vi "Test Camera Module.vi"(8 "error in (no error)":errorcluster) -> (0 "error in (no error) 2":errorcluster)   [LabVIEW 2015]
uses:
  <vilib>/userdefined/High Color/IMAQdx.ctl
  <vilib>/Utility/miscctls.llb/LVPointTypeDef.ctl
  <vilib>/vision/Image Controls.llb/IMAQ Image.ctl
panel:
  out "Status Queue":refnum<queue>
  out "Process Queue":refnum<queue>
  out "Live Queue":refnum<queue>
  in  "Grap image (trigger)":bool
  in  "stop grap":bool
  in  "Grap image":bool
  in  "Camera Connect":bool
  in  "Camera Disconnect":bool
  out "Status log":string
  in  "Camera ID":T1
  in  "Snap Image":bool
  in  "stop":bool
  out "Process Image":T2(plugin-control)
  # "Tests"
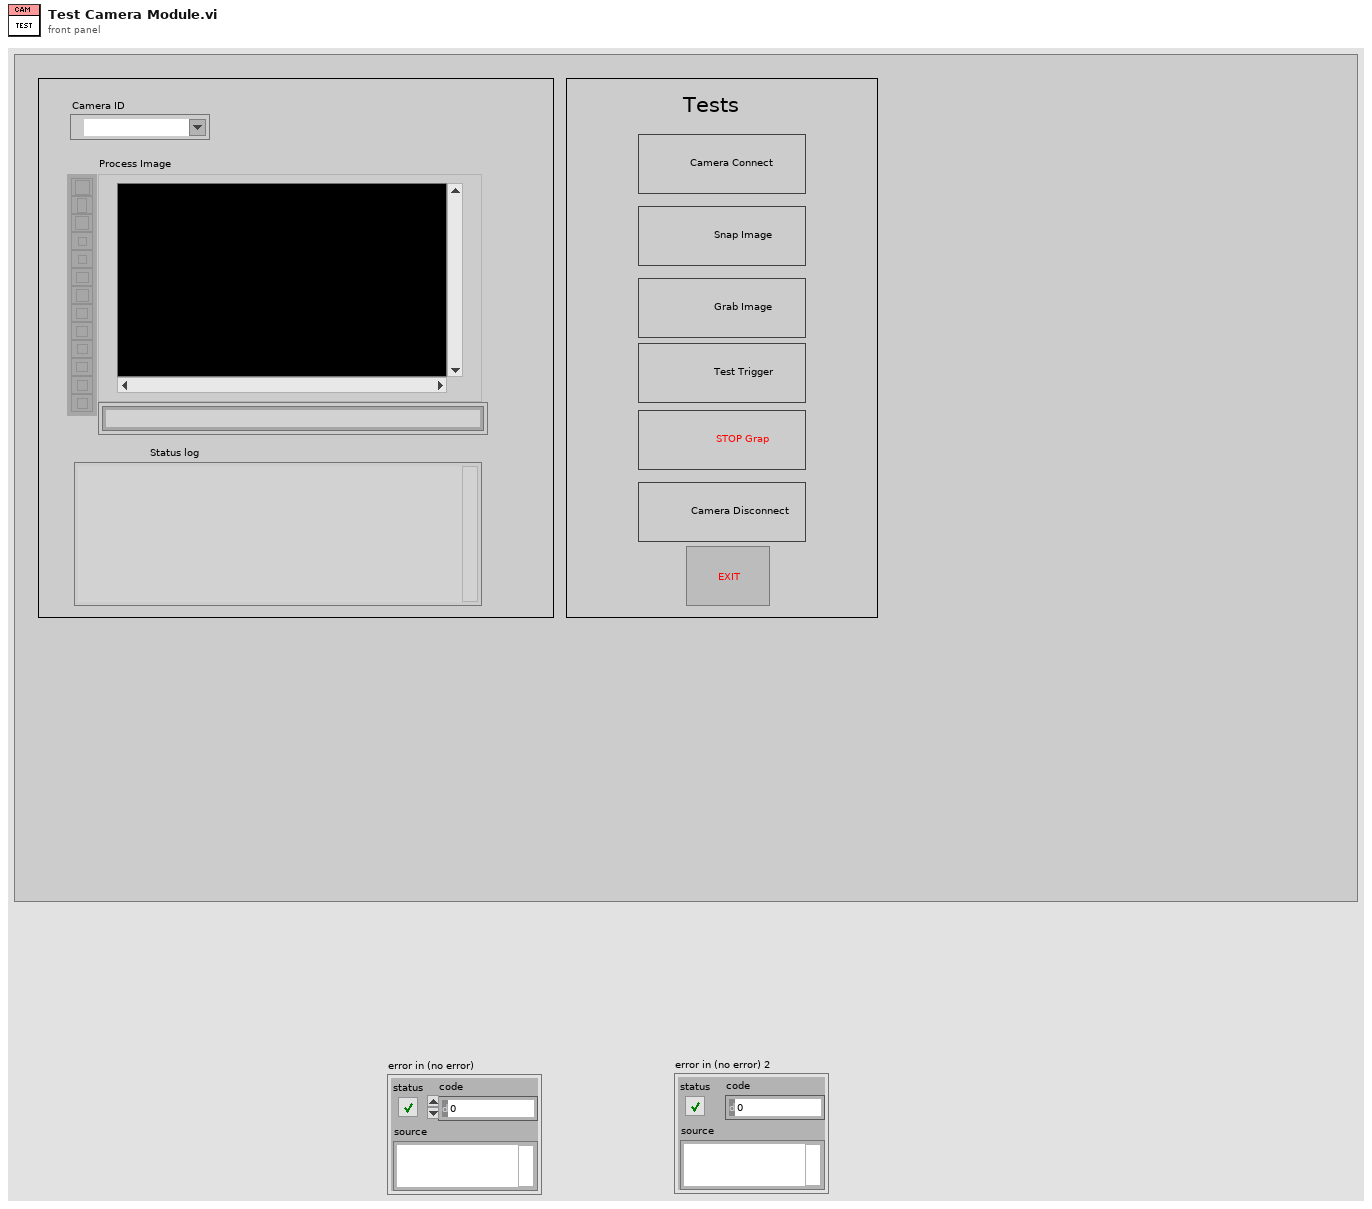
[diagram p1: front panel]
types:
  T1 = typedef "IMAQdx.ctl" = refnum<k21>
  T2 = typedef "IMAQ Image.ctl" = refnum<image>
  T3 = cluster{"Message":string, "Message Data":variant}
  T4 = typedef "LVPointTypeDef.ctl" = cluster{"Horizontal":i16, "Vertical":i16}
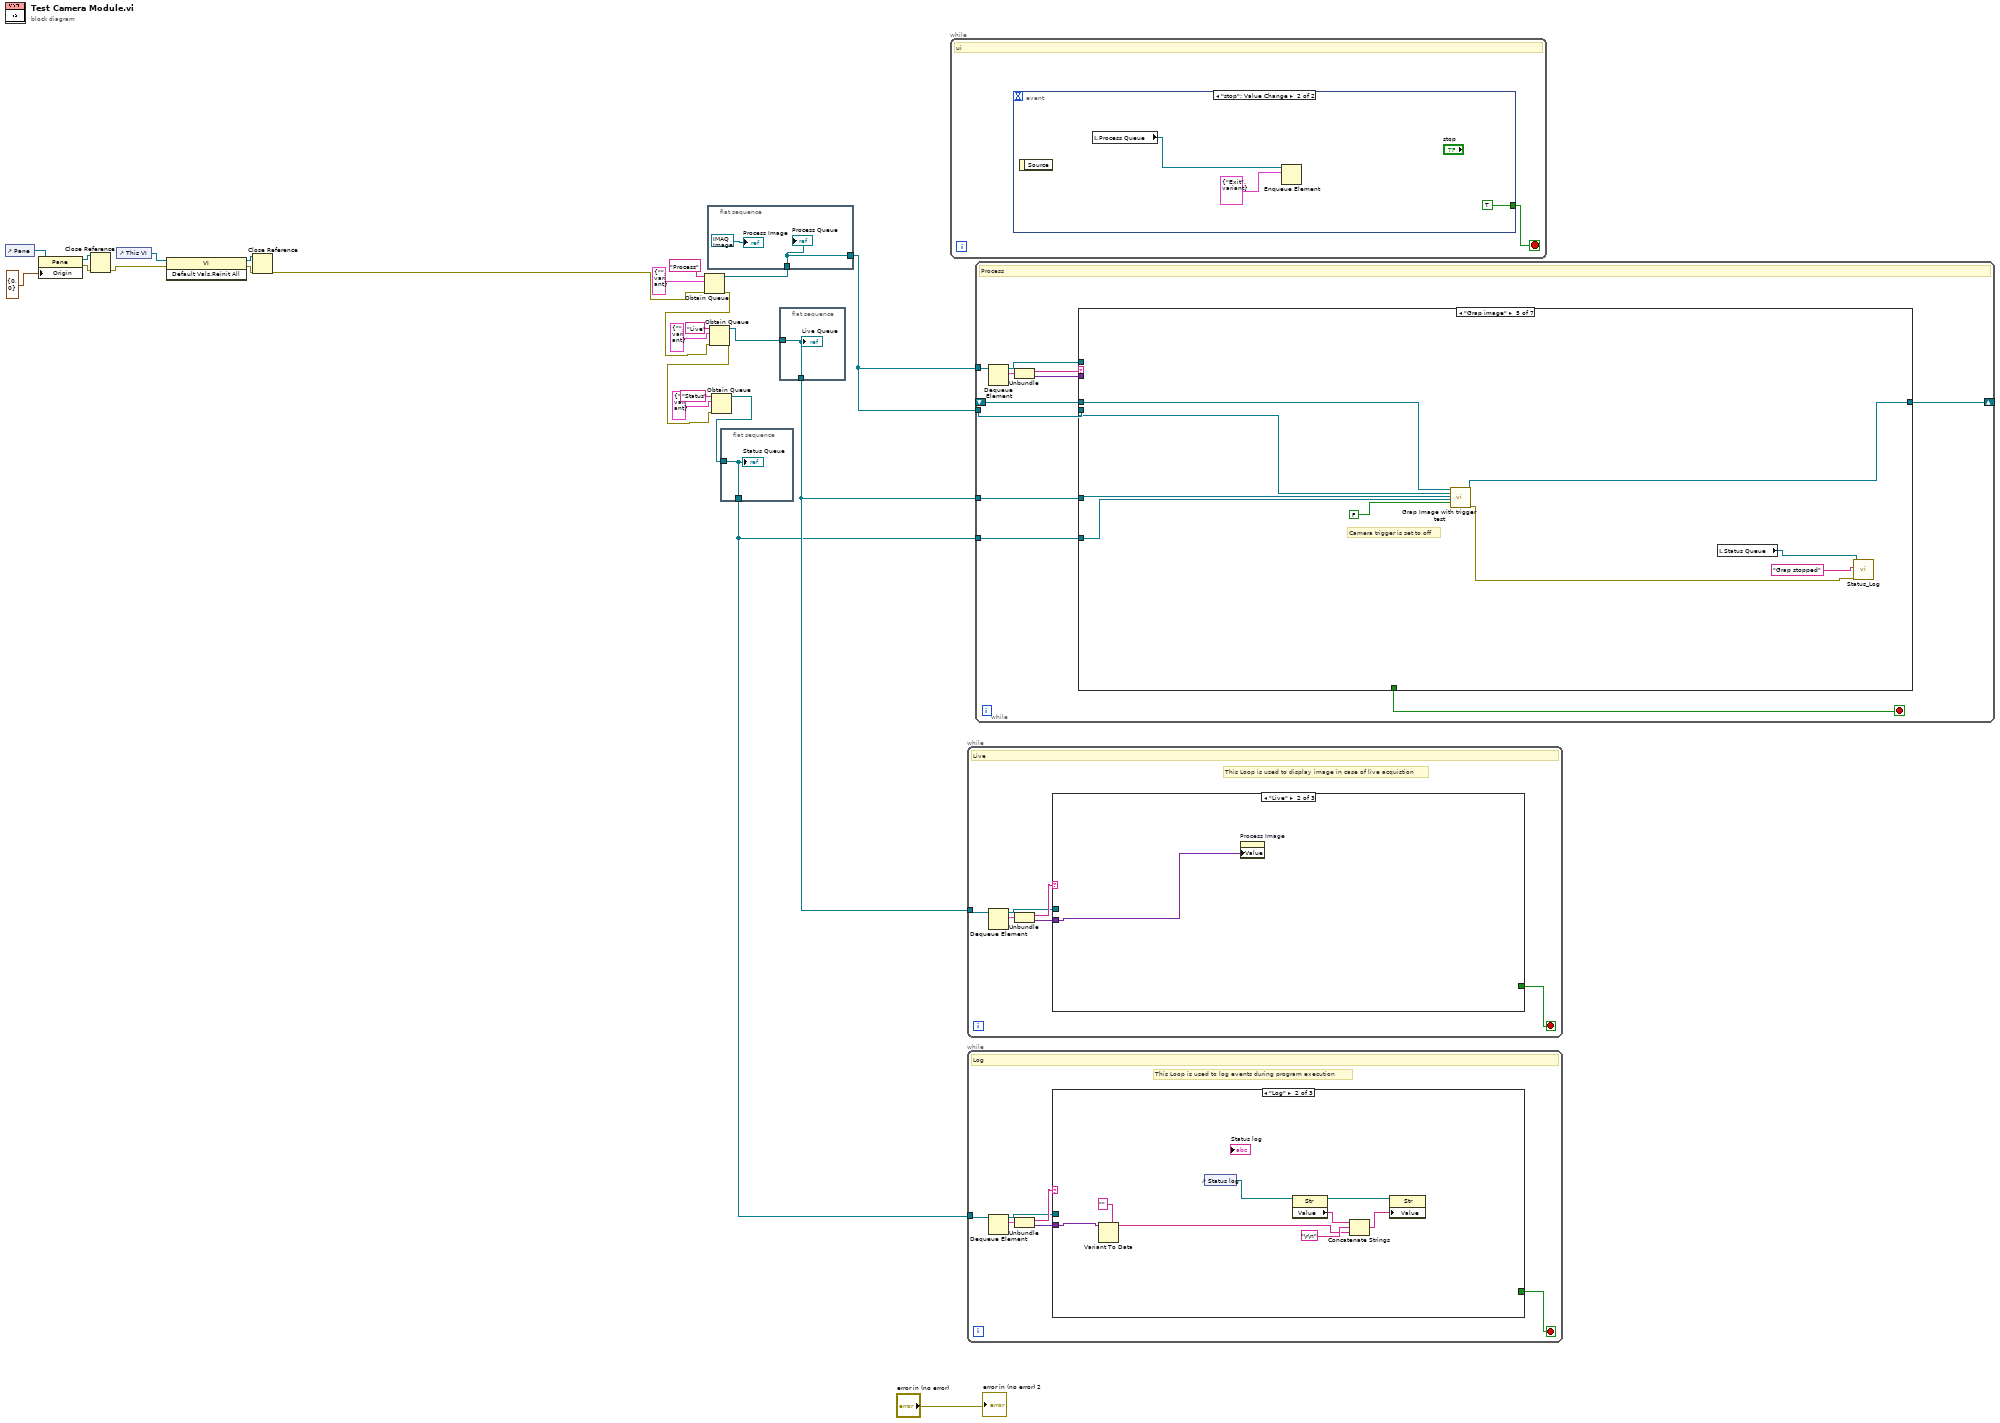
[diagram p0: block diagram]
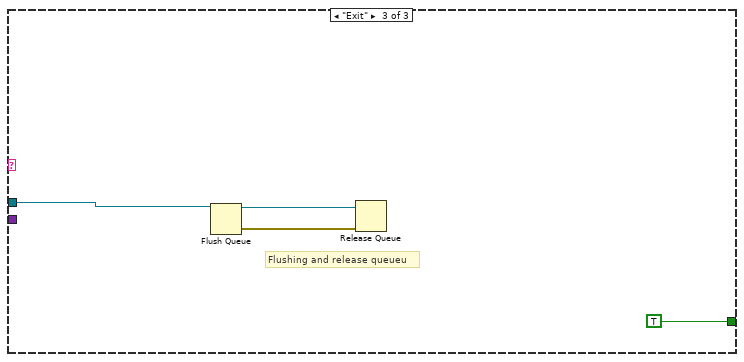
[diagram p3: hidden frame]
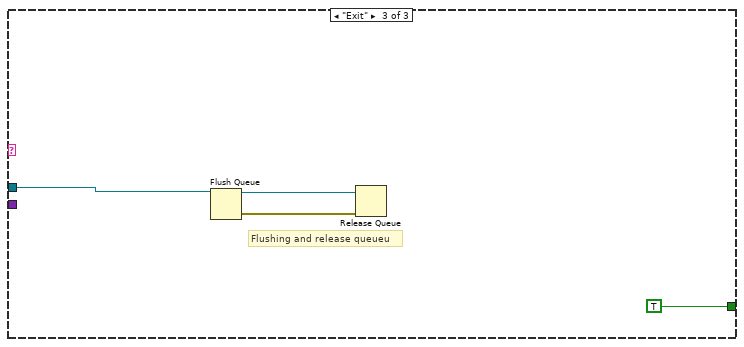
[diagram p5: hidden frame]
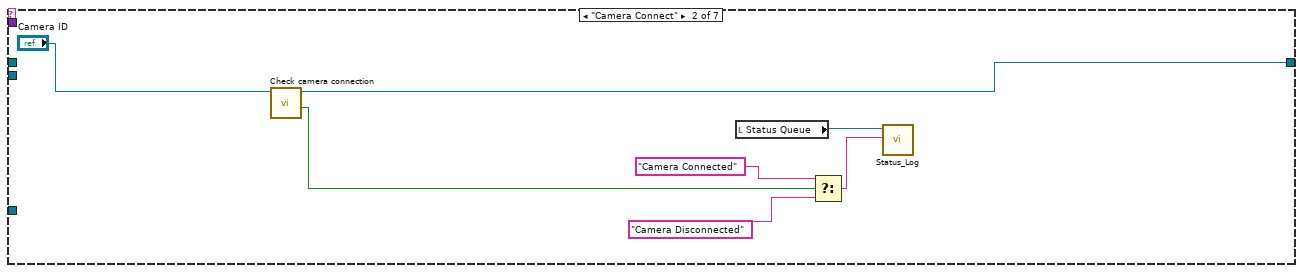
[diagram p7: hidden frame]
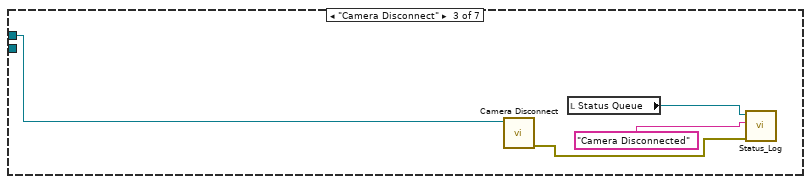
[diagram p8: hidden frame]
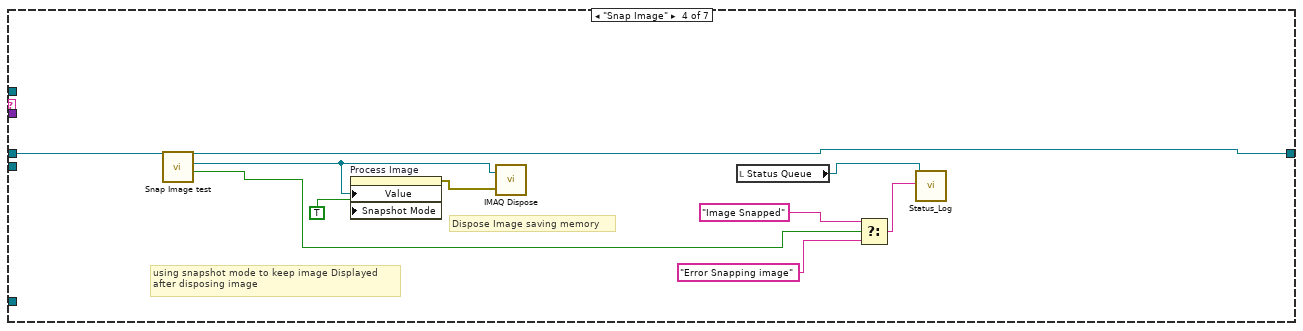
[diagram p9: hidden frame]
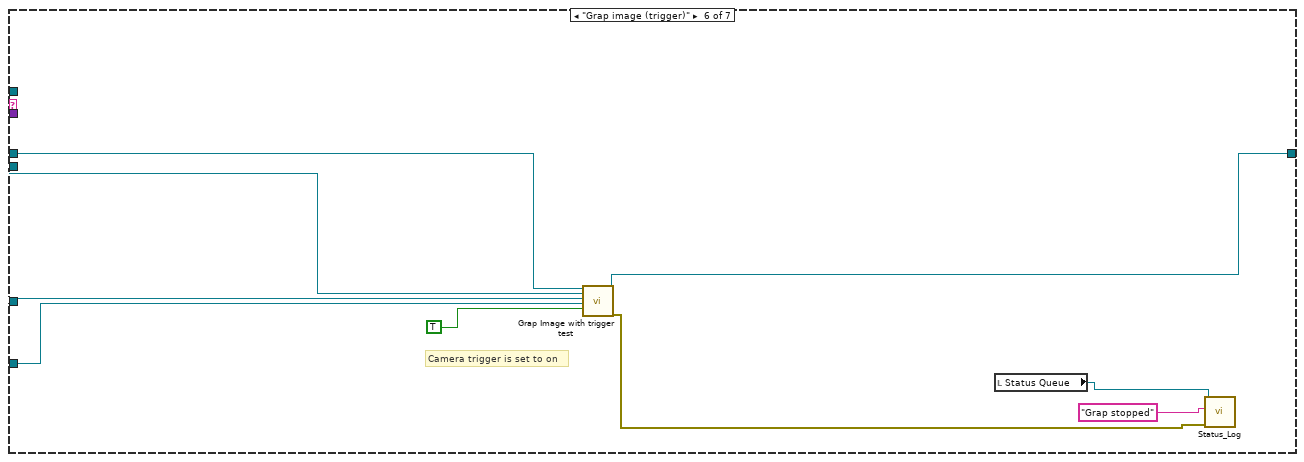
[diagram p10: hidden frame]
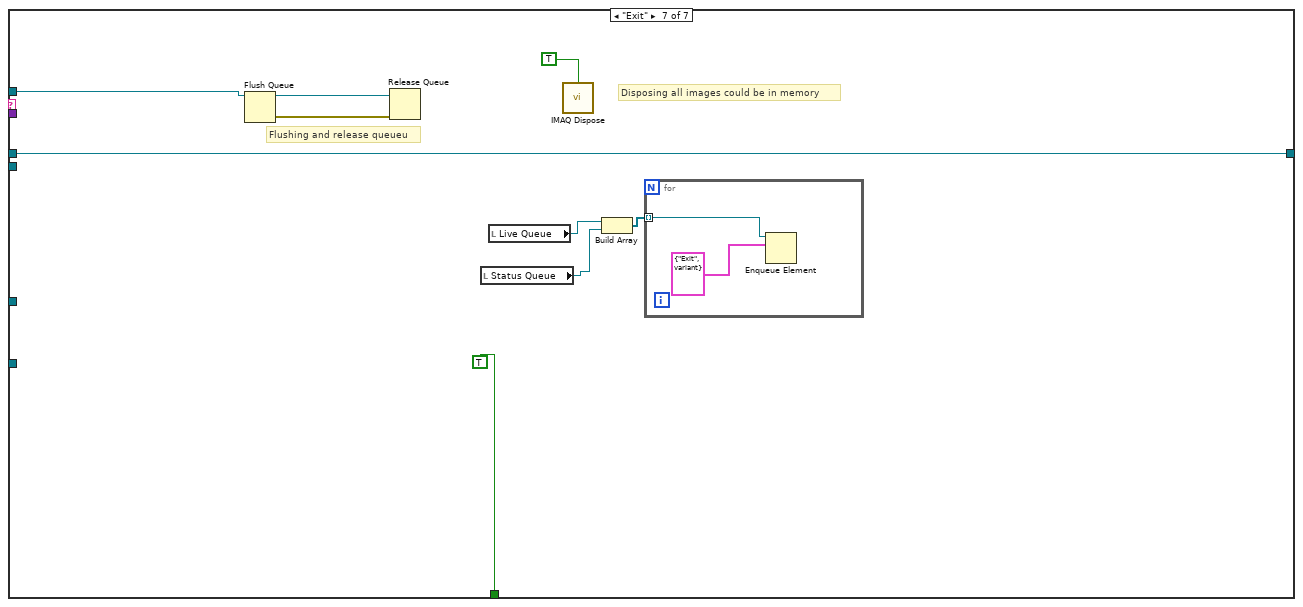
[diagram p11: hidden frame]
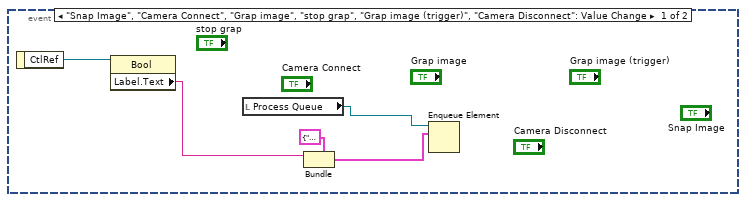
[diagram p12: hidden frame]
diagram:
  n1 = control-ref of="Pane"() -> (w17:refnum<vi>)
  n2 = property class="Pane"(reference=w17, "Origin"=T4 {"Horizontal"=0, "Vertical"=0}) -> (reference out=w19:refnum<vi>, error out=w20:errorcluster)  [unwired: 1 in]
  n3 = Close Reference(reference=w19, error in (no error)=w20) -> (error out=w16:errorcluster)
  n4 = control-ref of="This VI"() -> (w23:refnum<vi>)
  n5 = invoke class="VI" method="Default Vals.Reinit All"(reference=w23, error in=w16) -> (reference out=w21:refnum<vi>, error out=w22:errorcluster)  [unwired: 1 in, 1 out]
  n6 = Close Reference(reference=w21, error in (no error)=w22) -> (error out=w15:errorcluster)
  n7 = Obtain Queue(name (unnamed)="Process", element data type=T3 {"Message"="", "Message Data"=variant} ("Message Cluster"), error in (no error)=w15) -> (queue out=w13:refnum<queue>, error out=w6:errorcluster)  [unwired: 2 in, 1 out]
  n8 = flat-sequence {
    tunnel: w13 -> [w26]
    tunnel: [w26] -> w7
    frame #0 {
      "Process Queue" <- w26
      "Process Image" <- T2 refnum ("Process Image")
    }
  }
  n9 = Obtain Queue(name (unnamed)="Live", element data type=T3 {"Message"="", "Message Data"=variant} ("Message Cluster"), error in (no error)=w6) -> (queue out=w9:refnum<queue>, error out=w3:errorcluster)  [unwired: 2 in, 1 out]
  n10 = Obtain Queue(name (unnamed)="Status", element data type=T3 {"Message"="", "Message Data"=variant} ("Message Cluster"), error in (no error)=w3) -> (queue out=w2:refnum<queue>)  [unwired: 2 in, 2 out]
  n11 = flat-sequence {
    tunnel: w2 -> [w27]
    tunnel: [w27] -> w1
    frame #0 {
      "Status Queue" <- w27
    }
  }
  n12 = flat-sequence {
    tunnel: w9 -> [w28]
    tunnel: [w28] -> w8
    frame #0 {
      "Live Queue" <- w28
    }
  }
  n13 = while {
    stop <- w29 stop-if-true
    # "ui"
    n14 = event shown="[1] \"stop\": Value Change" {
      selector: _ -> [_ _]
      dyn-events: _ -> [_ _]
      timeout: _ -> [_ _]
      tunnel: [_ TRUE] -> w29
      event "Snap Image", "Camera Connect", "Grap image", "stop grap", "Grap image (trigger)", "Camera Disconnect": Value Change {
        n15 = event-data() -> ("CtlRef"=w32:refnum<vi>)  [unwired: 1 in]
        n16 = property class="Bool"(reference=w32) -> ("Label.Text"=w31:string)  [unwired: 1 in, 2 out]
        n17 = local read "Process Queue"() -> (w30:refnum<queue>)
        n18 = Bundle(cluster=T3 {"Message"="Update Module Data", "Message Data"=variant} ("element"), "Message"=w31) -> (w33:T3)  [unwired: 1 in]
        n19 = Enqueue Element(queue=w30, element=w33) -> ()  [unwired: 2 in, 3 out]
      }
      event "stop": Value Change {
        n20 = event-data() -> ()  [unwired: 1 in, 1 out]
        n21 = local read "Process Queue"() -> (w35:refnum<queue>)
        n22 = Enqueue Element(queue=w35, element=T3 {"Message"="Exit", "Message Data"=variant}) -> ()  [unwired: 2 in, 3 out]
      }
    }
  }
  n23 = while {
    tunnel: w8 -> [w42]
    stop <- w39 stop-if-true
    # "This Loop is used to display image in case of live acquistion"
    # "Live"
    n24 = Dequeue Element(queue=w42) -> (queue out=w38:refnum<queue>, element=w43:T3)  [unwired: 2 in, 2 out]
    n25 = Unbundle(w43) -> ("Message"=w41:string, "Message Data"=w40:variant)
    n26 = case shown="\"Live\"" w41 {
      tunnel: w40 -> [_ w44 _]
      tunnel: [_ _ TRUE] -> w39
      tunnel: w38 -> [_ _ w45]
      frame "False", Default {
      }
      frame "Live" {
        n27 = property on="Process Image" class="ImageControl"("Value"=w44) -> ()  [unwired: 2 in, 2 out]
      }
      frame "Exit" {
        # "Flushing and release queueu"
        n28 = Flush Queue(queue=w45) -> (queue out=w47:refnum<queue>, error out=w46:errorcluster)  [unwired: 1 in, 1 out]
        n29 = Release Queue(queue=w47, error in (no error)=w46) -> ()  [unwired: 1 in, 3 out]
      }
    }
  }
  n30 = while {
    tunnel: w1 -> [w53]
    stop <- w50 stop-if-true
    # "This Loop is used to log events during program execution"
    # "Log"
    n31 = Dequeue Element(queue=w53) -> (queue out=w49:refnum<queue>, element=w54:T3)  [unwired: 2 in, 2 out]
    n32 = Unbundle(w54) -> ("Message"=w52:string, "Message Data"=w51:variant)
    n33 = case shown="\"Log\"" w52 {
      tunnel: w51 -> [_ w57 _]
      tunnel: [_ _ TRUE] -> w50
      tunnel: w49 -> [_ _ w63]
      frame Default {
      }
      frame "Log" {
        n34 = Variant To Data(type="", Variant=w57) -> (data=w55:string)  [unwired: 1 in, 1 out]
        n35 = control-ref of="Status log"() -> (w58:refnum<vi>)
        n36 = property class="Str"(reference=w58) -> (reference out=w59:refnum<vi>, "Value"=w62:string)  [unwired: 1 in, 1 out]
        n37 = Concatenate Strings(w62, "\r\n", w55) -> (w60:string)
        n38 = property class="Str"(reference=w59, "Value"=w60) -> ()  [unwired: 1 in, 2 out]
      }
      frame "Exit" {
        # "Flushing and release queueu"
        n39 = Flush Queue(queue=w63) -> (queue out=w65:refnum<queue>, error out=w64:errorcluster)  [unwired: 1 in, 1 out]
        n40 = Release Queue(queue=w65, error in (no error)=w64) -> ()  [unwired: 1 in, 3 out]
      }
    }
  }
  n41 = while {
    tunnel: w7 -> [w77]
    tunnel: w7 -> [w73]
    shift-right: [w70] -> _
    shift-left: _ -> [w69]
    tunnel: w8 -> [w68]
    tunnel: w1 -> [w67]
    stop <- w71 stop-if-true
    # "Process"
    n42 = Dequeue Element(queue=w77) -> (queue out=w72:refnum<queue>, element=w76:T3)  [unwired: 2 in, 2 out]
    n43 = Unbundle(w76) -> ("Message"=w75:string, "Message Data"=w74:variant)
    n44 = case shown="\"Grap image\"" w75 {
      tunnel: w74 -> [_ _ _ _ _ _ _]
      tunnel: w73 -> [_ _ _ _ w103 w112 _]
      tunnel: w72 -> [_ _ _ _ _ _ w124]
      tunnel: [_ _ _ _ _ _ TRUE] -> w71
      tunnel: [w78 w85 _ w98 w107 w116 w125] -> w70
      tunnel: w69 -> [w78 _ w88 w99 w108 w117 w125]
      tunnel: w68 -> [_ _ _ _ w102 w111 _]
      tunnel: w67 -> [_ _ _ _ w101 w110 _]
      frame "False", Default {
      }
      frame "Camera Connect" {
        n45 = call "Check camera connection.vi"("Refnum in"="Camera ID") -> ("Connected ?"=w79:bool, "Refnum out"=w85:T1)  [unwired: 8 in, 1 out]
        n46 = local read "Status Queue"() -> (w80:refnum<queue>)
        n47 = Select(t="Camera Connected", s=w79, f="Camera Disconnected") -> (s? t:f=w81:string)
        n48 = call "Status_Log.vi"("String"=w81, "Status Queue"=w80) -> ()  [unwired: 9 in, 1 out]
      }
      frame "Camera Disconnect" {
        n49 = call "Camera Disconnect.vi"("Refnum in"=w88) -> ("error out"=w87:errorcluster)  [unwired: 10 in]
        n50 = local read "Status Queue"() -> (w86:refnum<queue>)
        n51 = call "Status_Log.vi"("error in (no error)"=w87, "String"="Camera Disconnected", "Status Queue"=w86) -> ()  [unwired: 8 in, 1 out]
      }
      frame "Snap Image" {
        # "using snapshot mode to keep image Displayed\nafter disposing image"
        # "Dispose Image saving memory"
        n52 = call "Snap Image test.vi"("Refnum in"=w99) -> ("Pass ?"=w94:bool, "Image Out"=w91:T2, "Refnum out"=w98:T1)  [unwired: 7 in, 1 out]
        n53 = property on="Process Image" class="ImageControl"("Value"=w91, "Snapshot Mode"=TRUE) -> (error out=w92:errorcluster)  [unwired: 2 in, 1 out]
        n54 = call "IMAQ Dispose"("Image"=w91, "error in (no error)"=w92) -> ()  [unwired: 4 in, 1 out]
        n55 = local read "Status Queue"() -> (w90:refnum<queue>)
        n56 = Select(t="Image Snapped", s=w94, f="Error Snapping image") -> (s? t:f=w95:string)
        n57 = call "Status_Log.vi"("String"=w95, "Status Queue"=w90) -> ()  [unwired: 9 in, 1 out]
      }
      frame "Grap image" {
        # "Camera trigger is set to off"
        n58 = call "Grap Image with trigger test.vi"("Refnum in"=w108, "Process Queueu"=w103, "Live Queue"=w102, "Status Queueu"=w101, "Trigger is on ?"=FALSE) -> ("Refnum out"=w107:T1, "error out"=w105:errorcluster)  [unwired: 12 in, 1 out]
        n59 = local read "Status Queue"() -> (w104:refnum<queue>)
        n60 = call "Status_Log.vi"("error in (no error)"=w105, "String"="Grap stopped", "Status Queue"=w104) -> ()  [unwired: 8 in, 1 out]
      }
      frame "Grap image (trigger)" {
        # "Camera trigger is set to on"
        n61 = call "Grap Image with trigger test.vi"("Refnum in"=w117, "Process Queueu"=w112, "Live Queue"=w111, "Status Queueu"=w110, "Trigger is on ?"=TRUE) -> ("Refnum out"=w116:T1, "error out"=w114:errorcluster)  [unwired: 12 in, 1 out]
        n62 = local read "Status Queue"() -> (w113:refnum<queue>)
        n63 = call "Status_Log.vi"("error in (no error)"=w114, "String"="Grap stopped", "Status Queue"=w113) -> ()  [unwired: 8 in, 1 out]
      }
      frame "Exit" {
        # "Flushing and release queueu"
        # "Disposing all images could be in memory"
        n64 = Flush Queue(queue=w124) -> (queue out=w123:refnum<queue>, error out=w122:errorcluster)  [unwired: 1 in, 1 out]
        n65 = Release Queue(queue=w123, error in (no error)=w122) -> ()  [unwired: 1 in, 3 out]
        n66 = local read "Status Queue"() -> (w121:refnum<queue>)
        n67 = local read "Live Queue"() -> (w120:refnum<queue>)
        n68 = call "IMAQ Dispose"("All Images? (No)"=TRUE) -> ()  [unwired: 5 in, 1 out]
        n69 = Build Array(w120, w121) -> (w119:refnum<queue>[])
        n70 = for {
          tunnel: w119 -> [w127] mode=indexing
          n71 = Enqueue Element(queue=w127, element=T3 {"Message"="Exit", "Message Data"=variant}) -> ()  [unwired: 2 in, 3 out]
        }
      }
    }
  }
  "error in (no error) 2" <- "error in (no error)"
